vi "PLL_Simple Phase and Frequency.vi"() -> ()   [LabVIEW 2019]
doc: "This VI adjusts both frequency and phase of one of the signals to be synchronized with the second one."
uses:
  <vilib>/measure/matone.llb/Extract Single Tone Information 1 Chan.vi
  <vilib>/measure/NI_MABase.lvlib
  <vilib>/Analysis/NI_AALPro.lvlib
  <vilib>/measure/NI_MAPro.lvlib
panel:
  out "Waveform Graph":waveform(dbl)[](graph)
  in  "stop":bool
  in  "Frequency [Hz]":dbl=10.0 format="%_6f"
  # "Overview:  This VI adjusts both frequency and phase of one of the signals to be synchronized with the second one.\nRequirements: LabVIEW 2012 (or compatible\nInstructions:\n1. Enter the desired signal frequency\n2. Run the VI\n3. Stop Execution"
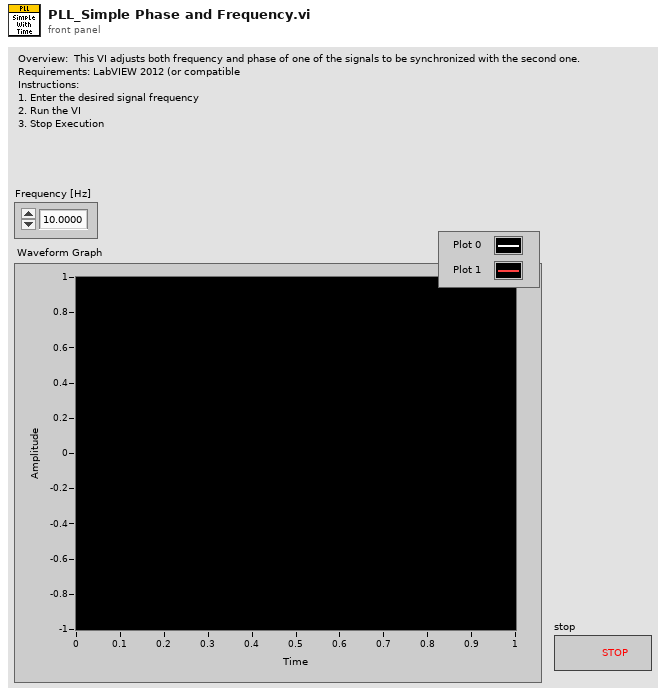
[diagram p1: front panel]
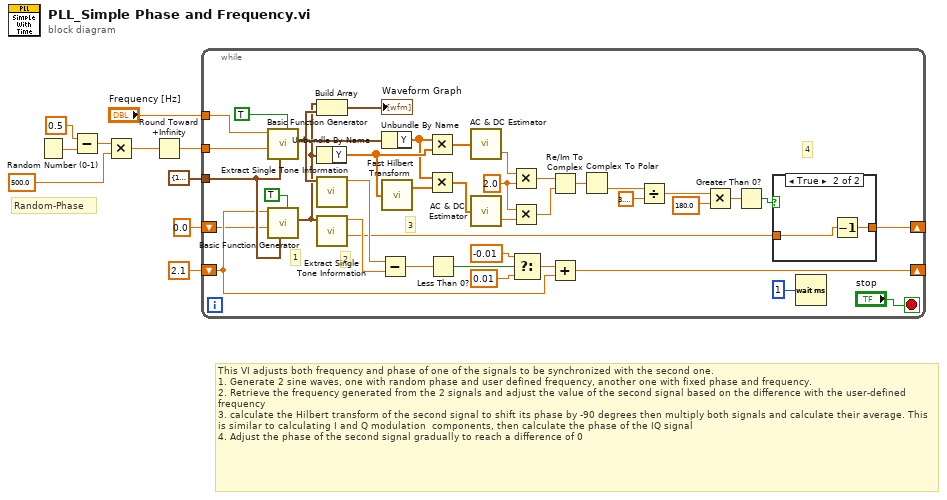
[diagram p0: block diagram]
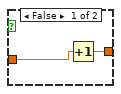
[diagram p2: hidden frame]
diagram:
  # "This VI adjusts both frequency and phase of one of the signals to be synchronized with the second one.\n1. Generate 2 sine waves, one with random phase and user defined frequency, another one with fixed phase and frequency.\n2. Retrieve the frequency generated from the 2 signals and adjust the value of the second signal based on the difference with the user-defined frequency\n3. calculate the Hilbert transform of the second signal to shift its phase by -90 degrees then multiply both signals and calculate their average. This is similar to calculating I and Q modulation  components, then calculate the phase of the IQ signal\n4. Adjust the phase of the second signal gradually to reach a difference of 0"
  # "Random-Phase"
  n1 = Random Number (0-1)() -> (number: 0 to 1=w7:dbl)
  n2 = Subtract(x=0.5, y=w7) -> (x-y=w5:dbl)
  n3 = Multiply(x=w5, y=500.0) -> (x*y=w3:dbl)
  n4 = Round Toward +Infinity(x=w3) -> (ceil(x): smallest int >= x=w2:dbl)
  n5 = while {
    tunnel: "Frequency [Hz]" -> [w44]
    tunnel: cluster{"Fs":dbl, "#s":dbl} {"Fs"=1000.0, "#s"=1000.0} ("sampling info") -> [w49]
    shift-right: [w20] -> _
    shift-left: 0.0 -> [w22]
    tunnel: w2 -> [w43]
    shift-right: [w36] -> _
    shift-left: 2.1 ("f") -> [w37]
    stop <- "stop" stop-if-true
    w14 = 2.0 ("x")
    # "4"
    # "3"
    # "2"
    # "1"
    n6 = call <vilib>:"Basic Function Generator.vi"("reset signal"=TRUE, "sampling info"=w49, "phase"=w43, "frequency"=w44) -> ("signal out"=w13:waveform(dbl))  [unwired: 5 in, 2 out]
    n7 = call <vilib>:"Basic Function Generator.vi"("reset signal"=TRUE, "sampling info"=w49, "phase"=w22, "frequency"=w37) -> ("signal out"=w12:waveform(dbl))  [unwired: 5 in, 2 out]
    n8 = Build Array(w12, w13) -> (→"Waveform Graph":waveform(dbl)[])
    n9 = Unbundle By Name(w12) -> ("Y"=w35:dbl[])
    n10 = call-poly <vilib>:"Extract Single Tone Information.vi"("time signal in"=w13) -> ("detected frequency"=w19:dbl)  [unwired: 5 in, 5 out]
    n11 = call-poly <vilib>:"Extract Single Tone Information.vi"("time signal in"=w12) -> ("detected phase (deg)"=w17:dbl, "detected frequency"=w18:dbl)  [unwired: 5 in, 4 out]
    n12 = Subtract(x=w19, y=w18) -> (x-y=w39:dbl)
    n13 = Unbundle By Name(w13) -> ("Y"=w33:dbl[])
    n14 = call <vilib>:"Fast Hilbert Transform.vi"("X"=w35) -> ("Hilbert{X}"=w34:dbl[])  [unwired: 1 out]
    n15 = Multiply(x=w33, y=w35) -> (x*y=w32:dbl[])
    n16 = Multiply(x=w33, y=w34) -> (x*y=w31:dbl[])
    n17 = Less Than 0?(x=w39) -> (x < 0?=w40:bool)
    n18 = call <vilib>:"AC & DC Estimator.vi"("Signal (V)"=w32) -> ("DC estimate (V)"=w15:dbl)  [unwired: 1 out]
    n19 = call <vilib>:"AC & DC Estimator.vi"("Signal (V)"=w31) -> ("DC estimate (V)"=w30:dbl)  [unwired: 1 out]
    n20 = Multiply(x=w15, y=w14) -> (x*y=w24:dbl)
    n21 = Multiply(x=w14, y=w30) -> (x*y=w23:dbl)
    n22 = Select(t=-0.01, s=w40, f=0.01) -> (s? t:f=w38:dbl)
    n23 = Re/Im To Complex(1:w23, 2:w24) -> (0:w25:cdb)
    n24 = Add(x=w38, y=w37) -> (x+y=w36:dbl)
    n25 = Complex To Polar(r * e^(i*theta)=w25) -> (theta=w26:dbl)  [unwired: 1 out]
    n26 = Divide(x=w26, y=3.141592653589793) -> (x/y=w28:dbl)
    n27 = Multiply(x=w28, y=180.0) -> (x*y=w16:dbl)
    n28 = Greater Than 0?(x=w16) -> (x > 0?=w21:bool)
    n29 = case shown="True" w21 {
      tunnel: w17 -> [w50 w52]
      tunnel: [w51 w53] -> w20
      frame False {
        n30 = Increment(x=w50) -> (x+1=w51:dbl)
      }
      frame True {
        n31 = Decrement(x=w52) -> (x-1=w53:dbl)
      }
    }
    n32 = Wait (ms)(milliseconds to wait=u32 1 ("millisecond multiple")) -> ()  [unwired: 1 out]
  }
